vi "Traçado_Gráfico_da_Função_SENO_com_uso_do_FORMULA_NODE.vi"() -> ()   [LabVIEW 2012]
panel:
  out "Waveform Chart":dbl(graph)
  in  "OK Button":bool
  out "Amplitude*SEN x":dbl
  out "Angulo em Graus":i32
  in  "Delay":u32
  in  "Amplitude":dbl(knob) scale=0.0..50.0
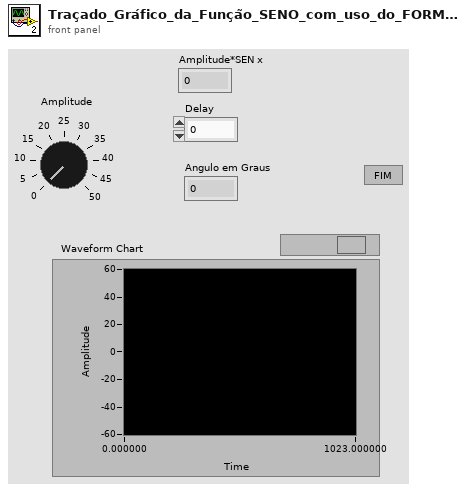
[diagram p1: front panel]
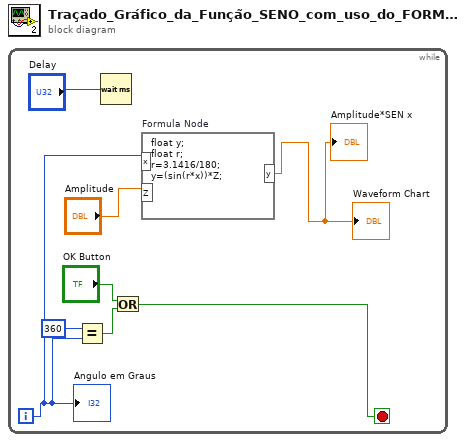
[diagram p0: block diagram]
diagram:
  n1 = while {
    i -> [w2]
    stop <- w4 stop-if-true
    n2 = Equal?(x=360, y=w2) -> (x = y?=w6:bool)
    n3 = Wait (ms)(milliseconds to wait="Delay") -> ()  [unwired: 1 out]
    n4 = Or(x="OK Button", y=w6) -> (x .or. y?=w4:bool)
    n5 = formula code="float y;\nfloat r;\nr=3.1416/180;\ny=(sin(r*x))*Z;"("Z"="Amplitude", "x"=w2) -> ("y"=→"Amplitude*SEN x" →"Waveform Chart":dbl)
    "Angulo em Graus" <- w2
  }
